vi "path.amd64.vi"() -> (0 "lib path":path)   [LabVIEW 2019, in "D2XX.lvlib" / "amd64.lvclass"]
uses:
  amd64.lvclass
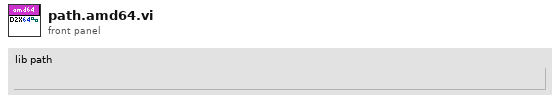
[diagram p1: front panel]
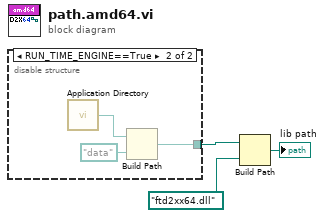
[diagram p0: block diagram]
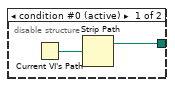
[diagram p2: hidden frame]
diagram:
  n1 = disable-structure shown="RUN_TIME_ENGINE==True" {
    disable-tunnel: [w4 w7] -> w1
    frame condition #0 (active) {
      n2 = Current VI's Path() -> (path=w5:path)
      n3 = Strip Path(path=w5) -> (stripped path=w4:path)  [unwired: 1 out]
    }
    frame condition #1 {
      n4 = call <vilib>:"Application Directory.vi"() -> ("Application Directory"=w6:path)
      n5 = Build Path(base path=w6, name or relative path=path "data") -> (appended path=w7:path)
    }
  }
  n6 = Build Path(base path=w1, name or relative path=path "ftd2xx64.dll") -> (appended path=→"lib path":path)
